vi "FGGA Serial Data Server & Recordingv3.1(serial_sim).vi"() -> ()   [LabVIEW 2014]
uses:
  <vilib>/Platform/TimedLoop/XDataNode/timing_clust.ctl
  <vilib>/Platform/TimedLoop/XDataNode/nitl_modes.ctl
  <vilib>/Platform/TimedLoop/XDataNode/wakeup.ctl
  C:/Program Files (x86)/National Instruments/LabVIEW 2014/examples/Data Communication/Network Streams/Simple Network Streams/support/Network Stream Command.ctl
  <vilib>/Utility/error.llb/whitespace.ctl
  <vilib>/Utility/tcp.llb/UDP Multicast Write-Only Open.vi
  <vilib>/Utility/tcp.llb/UDP Multicast Read-Only Open.vi
  <vilib>/Instr/_visa.llb/VISA Configure Serial Port (Instr).vi
  <vilib>/platform/TimedLoop/XDataNode/XDataNode.xnode
  <vilib>/Platform/TimedLoop/XDataNode/XDNodeRunTimeDep.lvlib
  <vilib>/Instr/_visa.llb/VISA Set IO Buffer Mask.ctl
  <vilib>/Instr/_visa.llb/VISA Flush IO Buffer Mask.ctl
panel:
  out "MFC":dbl[](array[numeric])
  out "FGGA restart":bool
  out "V4":bool
  out "V3":bool
  out "V2":bool
  out "V1":bool
  out "error out 2":errorcluster
  out "error out":errorcluster
  in  "MFC_1 SLPM set value":dbl
  out "Value Read":string
  out "status":bool
  in  "VISA resource name":refnum<visa-resource-name>="ASRL3::INSTR"
  in  "timeout (10sec) 2":u32=3000
  out "Labview_Viewer_UDP_Error_Out":errorcluster
  in  "Clear Display\nErrors":bool
  out "Data Processing":bool
  out "TCP Binary Packet":string
  in  "Time Stamp\nOffset":u32=1
  out "Data String":string
  out "UDP_ACSII_Out":string
  out "Serial error out":errorcluster
  out "SEPTIC TCP Error Out":errorcluster
  out "TCP packet\nSend To SEPTIC":bool
  out "FISH TCP Error Out":errorcluster
  out "TCP packet\nSend To FISH":bool
  out "UDP_Pack_num":u32
  out "UDP_Out Status":bool
  out "UDP_Out_Error Out":errorcluster
  out "UDP_In":string
  out "UDP_In_Error":errorcluster
  in  "Flight Number":string
  out "Data Array":string[](array[string])
  out "RAW DATA":string
  in  "stop":bool
  in  "timeout (10sec)":u32=1500
  in  "VISA resource name":refnum<visa-resource-name>="ASRL7::INSTR"
  out "Number of times \nRead time out":u32
  out "Loop count":i32
  # "Date"
  # "Time"
  # "CH4"
  # "CO2"
  # "H2O"
  # "Cell Pressure"
  # "Cell Temperature"
  # "Spectral Flag"
  # "Ring Down Time (Laser A)"
  # "Ring Down Time (Laser B)"
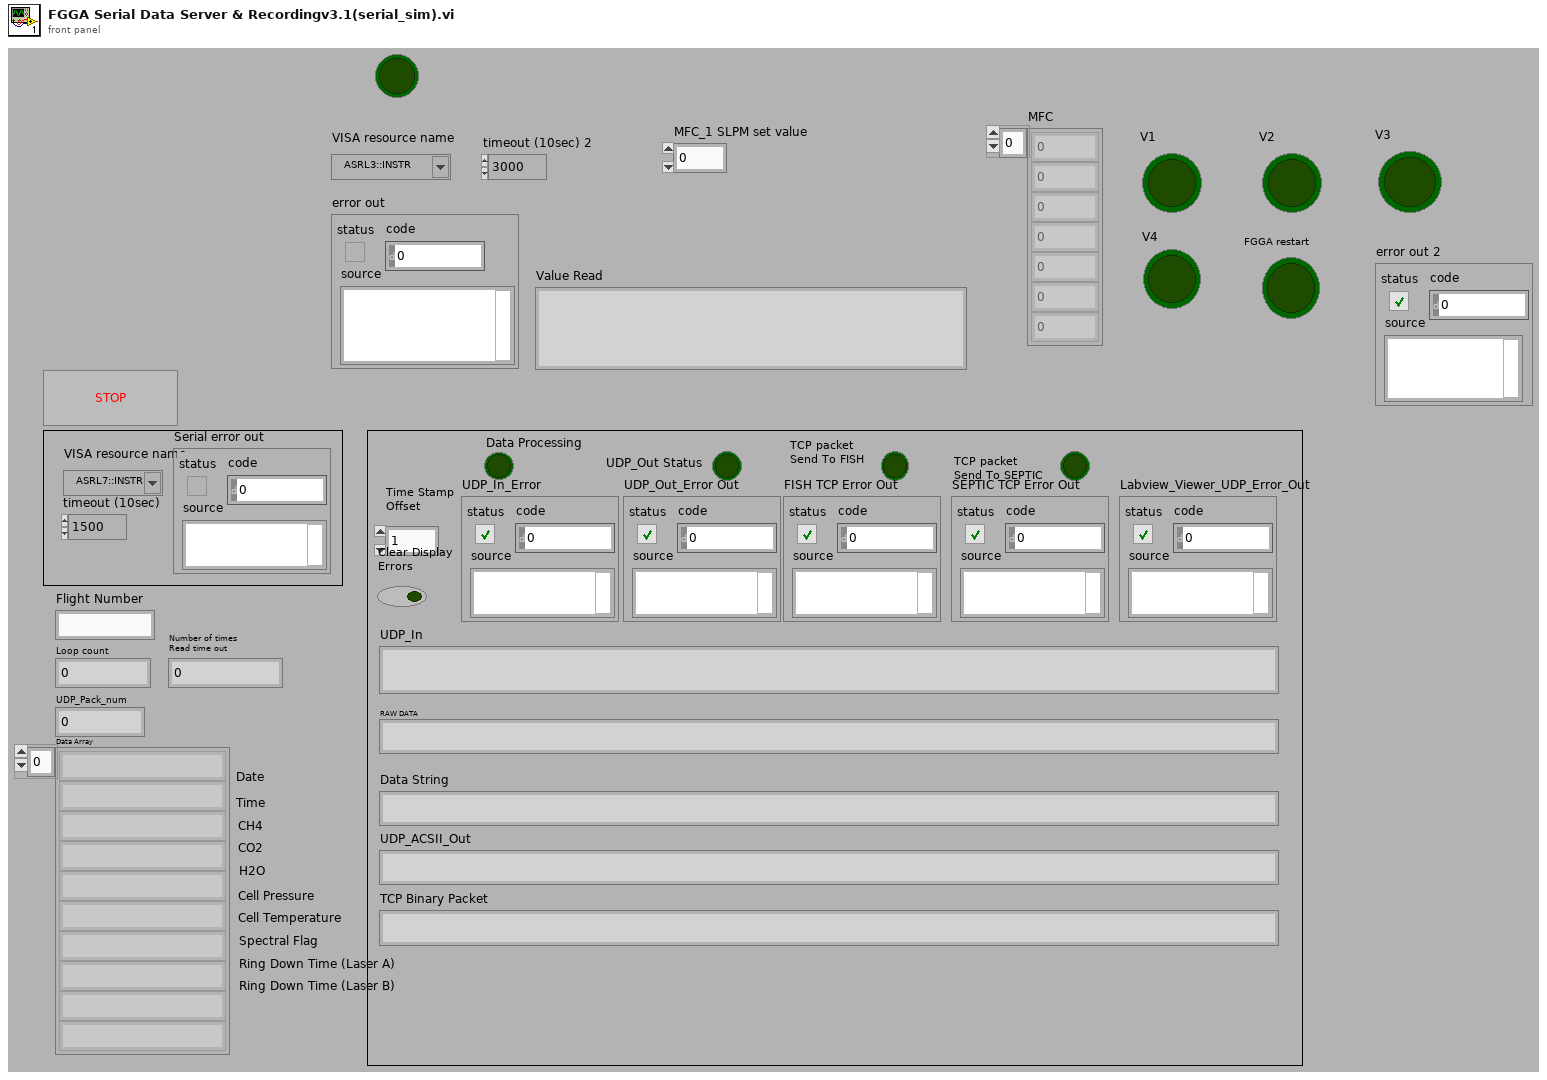
[diagram p1: front panel]
types:
  T1 = typedef "VISA Flush IO Buffer Mask.ctl" = u16
  T2 = typedef "VISA Set IO Buffer Mask.ctl" = u16
  T3 = typedef "Network Stream Command.ctl" = cluster{"Message":string, "Message Data":variant}
  T4 = typedef "XDNodeRunTimeDep.lvlib/timing_clust.ctl" = cluster{"Expected End [f-1]":u64, "Actual End [f-1]":u64, "Finished Late? [f-1]":bool, "Expected End [i-1]":u64, "Actual End [i-1]":u64, "Finished Late? [i-1]":bool, "Expected Start [i]":u64, "Actual Start [i]":u64, "Expected Start [f]":u64, "Actual Start [f]":u64, "Source Name":string, "Structure Name":string, "Period":i64, "Deadline":i64, "Offset":i64, "Start":i64, "Priority":i32, "Timeout":i32, "Mode":T5, "Wakeup Reason":T6, "Error":errorcluster, "Source Type":string, "Secondary Source Type":string, "Global End Time":u64, "Global Start Time":u64, "Frame Duration":u64, "Iteration Duration":u64, "Assigned CPU":i32, "I/O Scan Engine Mode":u32}
  T5 = typedef "XDNodeRunTimeDep.lvlib/nitl_modes.ctl" = enum32{"No Change", "Process missed periods, maintain original phase", "Discard missed periods, maintain original phase", "Process missed periods, ignore original phase", "Discard missed periods, ignore original phase"}
  T6 = typedef "XDNodeRunTimeDep.lvlib/wakeup.ctl" = enum32{"Normal", "Aborted", "Asynchronous wakeup", "Timing source error", "Timed loop error", "Timeout"}
  T7 = typedef "whitespace.ctl" = u16
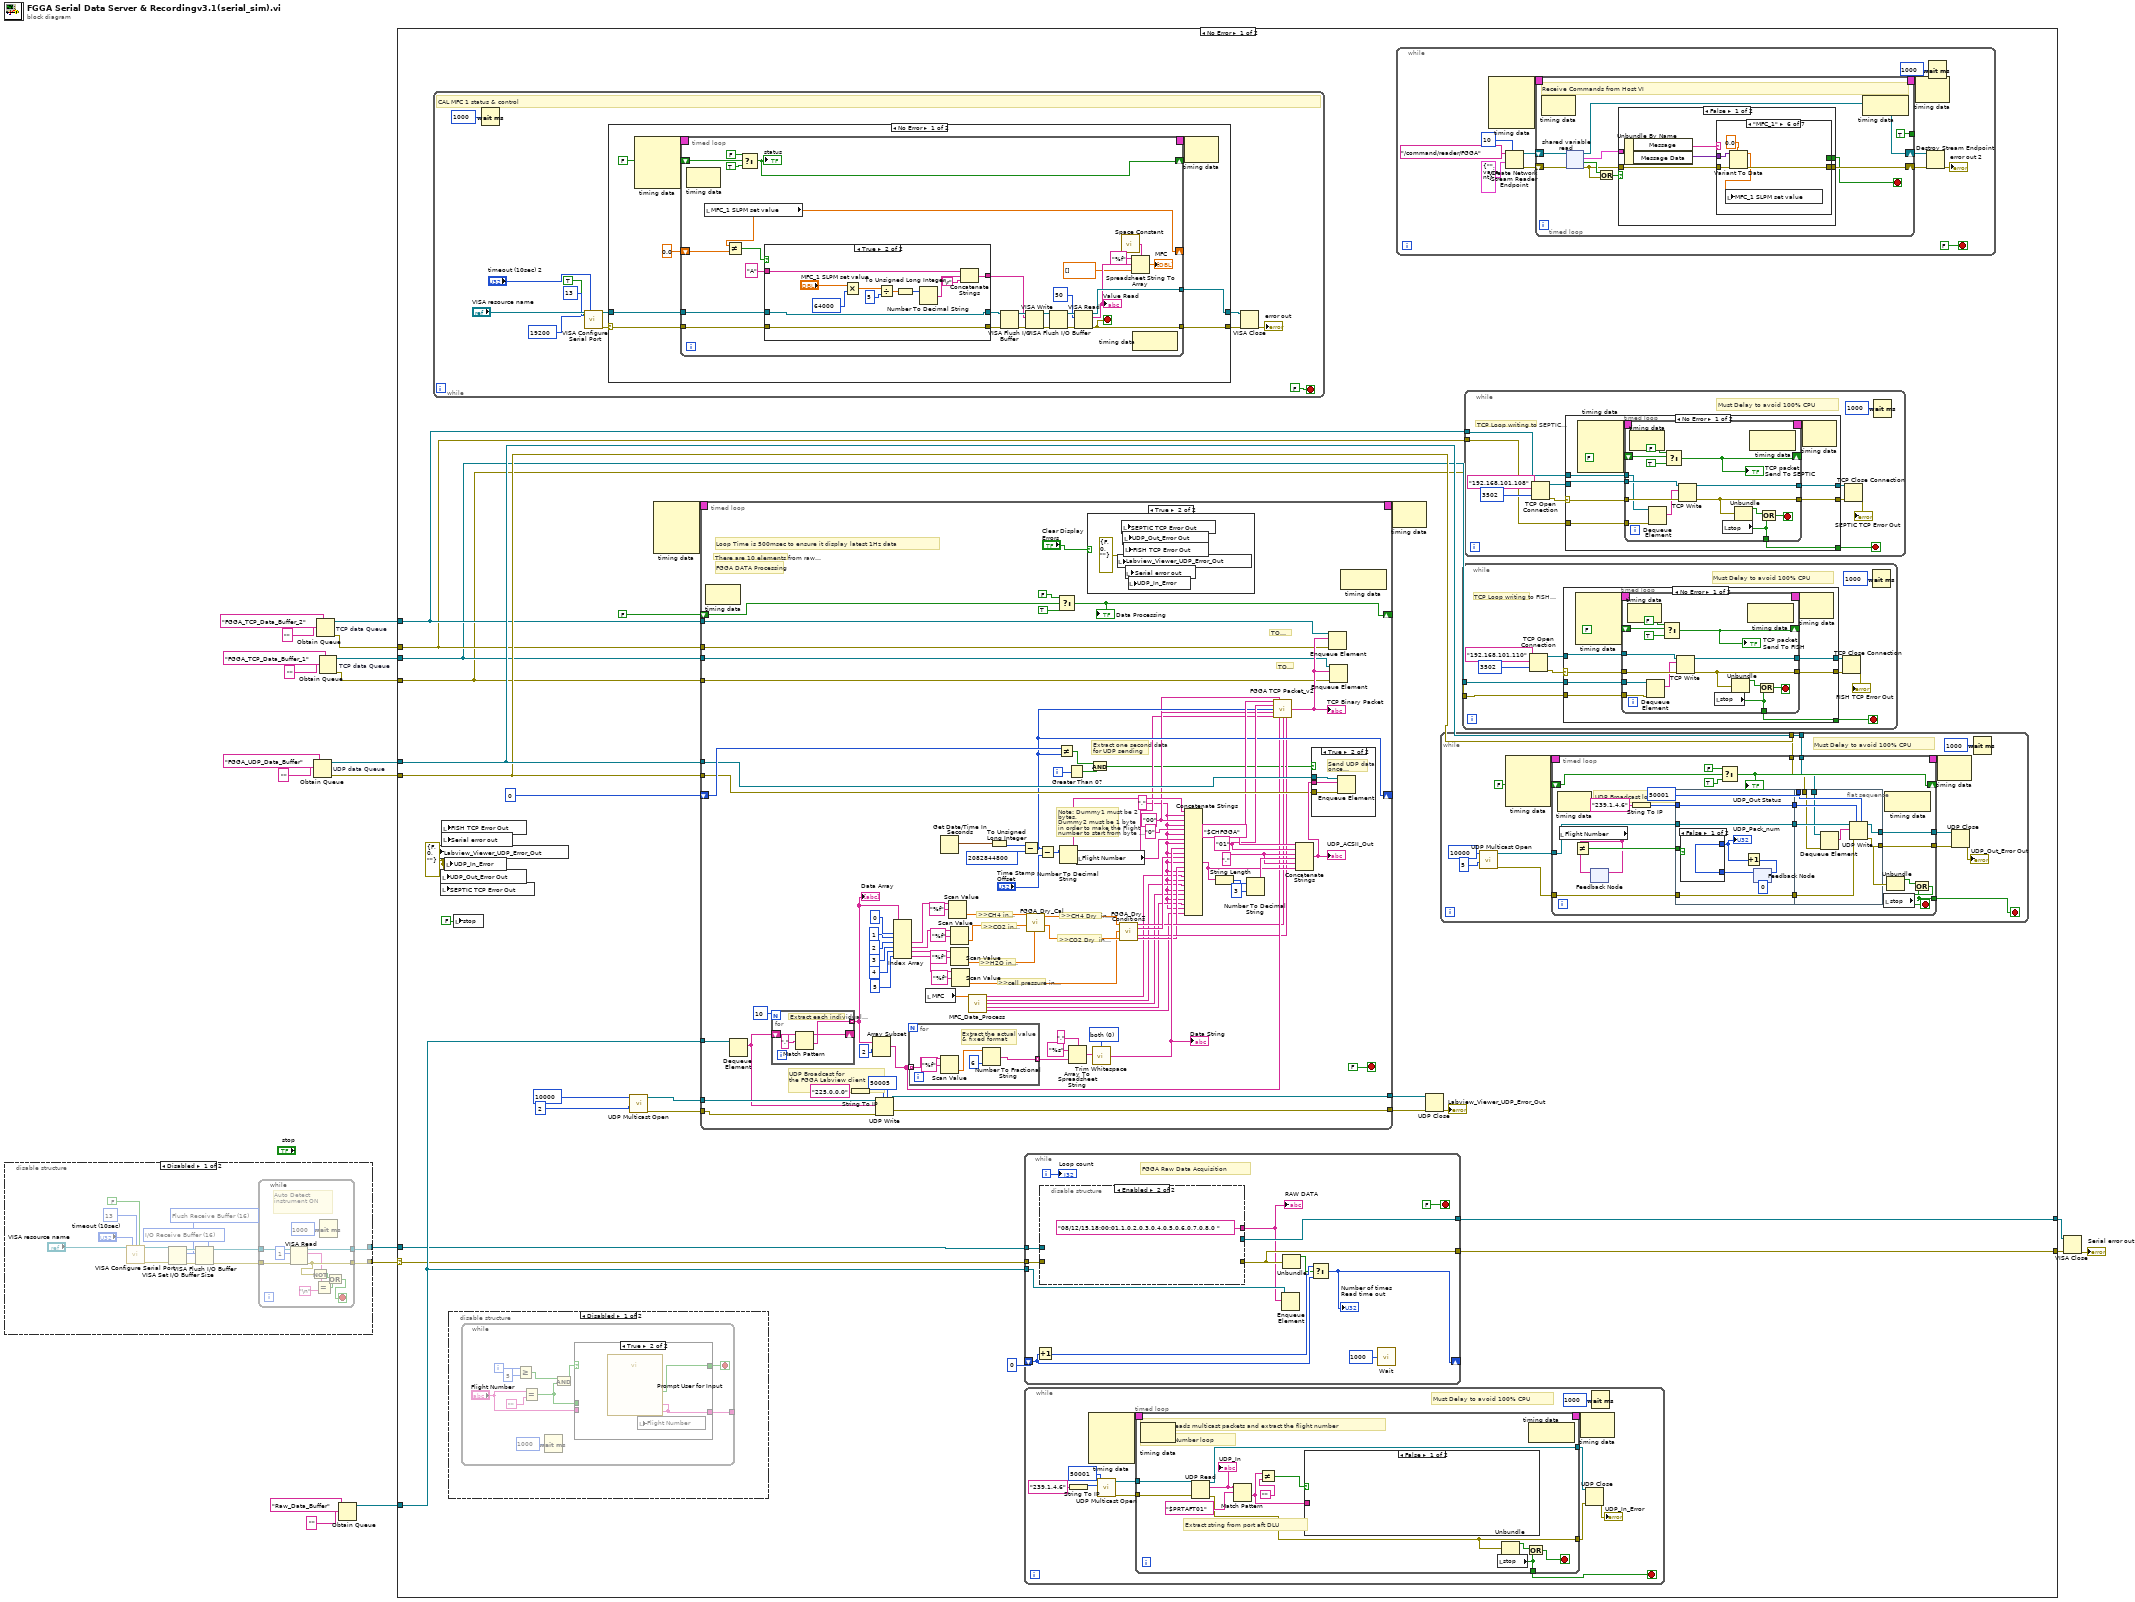
[diagram p0: block diagram]
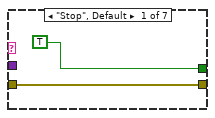
[diagram p3: hidden frame]
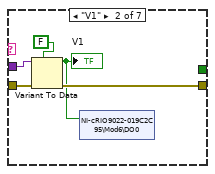
[diagram p4: hidden frame]
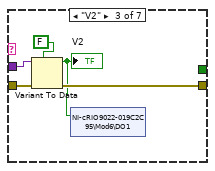
[diagram p5: hidden frame]
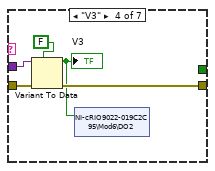
[diagram p6: hidden frame]
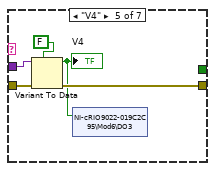
[diagram p7: hidden frame]
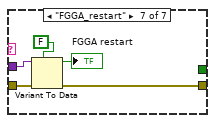
[diagram p8: hidden frame]
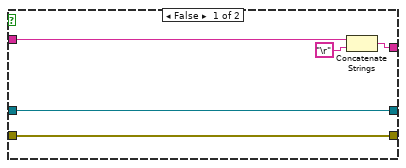
[diagram p10: hidden frame]
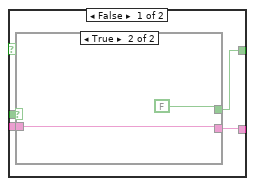
[diagram p12: hidden frame]
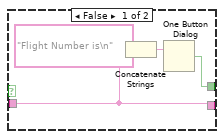
[diagram p13: hidden frame]
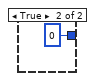
[diagram p15: hidden frame]
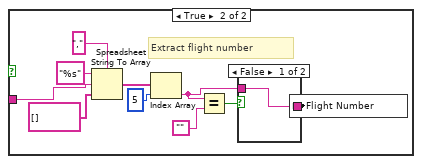
[diagram p16: hidden frame]
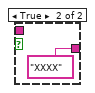
[diagram p17: hidden frame]
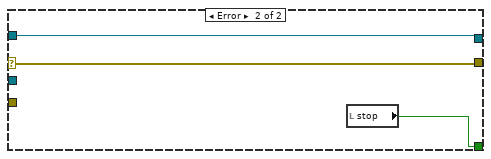
[diagram p18: hidden frame]
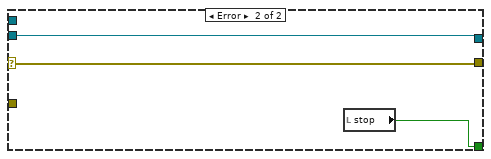
[diagram p19: hidden frame]
diagram:
  n1 = disable-structure shown="Disabled" {
    disable-tunnel: [w22 _] -> w2
    disable-tunnel: [w21 _] -> w1
    frame Disabled {
      w27 = T1 16 items=["Flush Receive Buffer"=16, "Write Transmit Buffer to Device"=32, "Flush Receive Buffer (No I/O)"=64, "Flush Transmit Buffer"=128] ("Mask")
      w28 = T2 16 items=["I/O Receive Buffer"=16, "I/O Transmit Buffer"=32, "I/O Receive and Transmit Buffer"=48] ("Mask")
      n2 = call-poly "VISA Configure Serial Port"("VISA resource name"="VISA resource name", "timeout (10sec)"="timeout (10sec)", "termination char\n(0xA = '\\n' = LF)"=u8 13 ("termination char\n(0xA = '\\n' = LF)"), "Enable Termination\nChar (T)"=FALSE ("Enable Termination\nChar (T)")) -> ("VISA resource name out"=w26:refnum<visa-resource-name>, "error out"=w25:errorcluster)  [unwired: 10 in]
      n3 = VISA Set I/O Buffer Size(VISA resource name=w26, mask (16)=w28, error in (no error)=w25) -> (VISA resource name out=w29:refnum<visa-resource-name>, error out=w30:errorcluster)  [unwired: 1 in]
      n4 = VISA Flush I/O Buffer(VISA resource name=w29, mask (16)=w27, error in (no error)=w30) -> (VISA resource name out=w24:refnum<visa-resource-name>, error out=w23:errorcluster)
      n5 = while {
        tunnel: w24 -> [w45]
        tunnel: w23 -> [w44]
        tunnel: [w42] -> w22
        tunnel: [w41] -> w21
        stop <- w36 stop-if-true
        # "Auto Detect\ninstrument ON"
        n6 = VISA Read(VISA resource name=w45, byte count=u32 1, error in (no error)=w44) -> (VISA resource name out=w41:refnum<visa-resource-name>, read buffer=w39:string, error out=w42:errorcluster)  [unwired: 1 out]
        n7 = Not(x=w42) -> (.not. x?=w38:bool)
        n8 = Equal?(x=w39, y="\n") -> (x = y?=w37:bool)
        n9 = Wait (ms)(milliseconds to wait=u32 1000) -> ()  [unwired: 1 out]
        n10 = Or(x=w38, y=w37) -> (x .or. y?=w36:bool)
      }
    }
    frame Enabled {
    }
  }
  n11 = Obtain Queue "UDP data Queue"(name (unnamed)="FGGA_UDP_Data_Buffer", element data type="") -> (queue out=w12:refnum<queue>, error out=w11:errorcluster)  [unwired: 3 in, 1 out]
  n12 = Obtain Queue "TCP data Queue"(name (unnamed)="FGGA_TCP_Data_Buffer_2", element data type="") -> (queue out=w6:refnum<queue>, error out=w5:errorcluster)  [unwired: 3 in, 1 out]
  n13 = Obtain Queue "TCP data Queue"(name (unnamed)="FGGA_TCP_Data_Buffer_1", element data type="") -> (queue out=w4:refnum<queue>, error out=w3:errorcluster)  [unwired: 3 in, 1 out]
  n14 = Obtain Queue(name (unnamed)="Raw_Data_Buffer", element data type="") -> (queue out=w18:refnum<queue>)  [unwired: 3 in, 2 out]
  n15 = case shown="No Error" w2 {
    selector: w2 -> [w46 w545]
    tunnel: w1 -> [w47 w546]
    tunnel: [w69 w546] -> w15
    tunnel: [w70 w545] -> w16
    tunnel: w18 -> [w65 _]
    tunnel: w12 -> [w63 _]
    tunnel: w11 -> [w62 _]
    tunnel: w6 -> [w61 _]
    tunnel: w5 -> [w60 _]
    tunnel: w4 -> [w59 _]
    tunnel: w3 -> [w58 _]
    frame No Error {
      w49 = errorcluster {"status"=FALSE, "code"=0, "source"=""} ("UDP Error Out")
      n16 = while {
        stop <- FALSE stop-if-true
        # "CAL MFC 1 status & control"
        n17 = Wait (ms)(milliseconds to wait=u32 1000) -> ()  [unwired: 1 out]
        n18 = call-poly "VISA Configure Serial Port"("VISA resource name"="VISA resource name", "timeout (10sec)"="timeout (10sec) 2", "termination char\n(0xA = '\\n' = LF)"=u8 13 ("termination char\n(0xA = '\\n' = LF)"), "Enable Termination\nChar (T)"=TRUE ("Enable Termination\nChar (T)"), "baud rate (9600)"=u32 19200) -> ("VISA resource name out"=w148:refnum<visa-resource-name>, "error out"=w144:errorcluster)  [unwired: 9 in]
        n19 = case shown="No Error" w144 {
          selector: w144 -> [w155 w205]
          tunnel: w148 -> [w156 w206]
          tunnel: [w154 w206] -> w147
          tunnel: [w153 w205] -> w146
          frame No Error {
            n20 = node-c288() -> (w151:T4)  [unwired: 4 in]
            n21 = timed-loop {
              tunnel: w156 -> [w179]
              tunnel: w155 -> [w177]
              tunnel: [w170] -> w154
              tunnel: [w165] -> w153
              shift-right: [w166] -> _
              shift-left: FALSE -> [w169]
              timing: w151 -> [_]
              timing-out: [_] -> w150
              shift-right: [w157] -> _
              shift-left: 0.0 -> [w159]
              stop <- w165 stop-if-true
              n22 = node-c288() -> ()  [unwired: 1 in, 1 out]
              n23 = local read "MFC_1 SLPM set value"() -> (w157:dbl)
              n24 = Not Equal?(x=w157, y=w159) -> (x != y?=w158:bool)
              n25 = Select(t=FALSE, s=w169, f=TRUE) -> (s? t:f=w166:bool)
              "status" <- w166
              n26 = case shown="True" w158 {
                tunnel: w179 -> [w187 w202]
                tunnel: [w187 w202] -> w178
                tunnel: w177 -> [w186 w201]
                tunnel: [w186 w201] -> w176
                tunnel: "A" -> [w190 w194]
                tunnel: [w188 w191] -> w174
                frame False {
                  n27 = Concatenate Strings(w190, "\r") -> (w188:string)
                }
                frame True {
                  n28 = Multiply(x="MFC_1 SLPM set value", y=u32 64000) -> (x*y=w198:dbl)
                  n29 = Divide(x=w198, y=u32 5) -> (x/y=w196:dbl)
                  n30 = To Unsigned Long Integer(number=w196) -> (unsigned 32bit integer=w195:u32)
                  n31 = Number To Decimal String(number=w195) -> (decimal integer string=w193:string)  [unwired: 1 in]
                  n32 = Concatenate Strings(w194, w193, "\r") -> (w191:string)
                }
              }
              n33 = VISA Flush I/O Buffer(VISA resource name=w178, error in (no error)=w176) -> (VISA resource name out=w181:refnum<visa-resource-name>, error out=w180:errorcluster)  [unwired: 1 in]
              n34 = VISA Write(VISA resource name=w181, write buffer=w174, error in (no error)=w180) -> (VISA resource name out=w173:refnum<visa-resource-name>, error out=w172:errorcluster)  [unwired: 1 out]
              n35 = VISA Flush I/O Buffer(VISA resource name=w173, error in (no error)=w172) -> (VISA resource name out=w183:refnum<visa-resource-name>, error out=w182:errorcluster)  [unwired: 1 in]
              n36 = VISA Read(VISA resource name=w183, byte count=u32 50, error in (no error)=w182) -> (VISA resource name out=w170:refnum<visa-resource-name>, read buffer=w164:string, error out=w165:errorcluster)  [unwired: 1 out]
              "Value Read" <- w164
              n37 = call <vilib>:"Space Constant.vi"() -> ("String"=w163:string)
              n38 = Spreadsheet String To Array(delimiter (Tab)=w163, format string="%f", spreadsheet string=w164, array type (2D Dbl)=dbl[] []) -> (array=→"MFC":dbl[])
              n39 = node-c288() -> ()  [unwired: 1 in, 1 out]
            }
            n40 = node-c288(w150) -> ()  [unwired: 1 out]
          }
          frame Error {
          }
        }
        n41 = VISA Close(VISA resource name=w147, error in (no error)=w146) -> (error out=→"error out":errorcluster)
      }
      n42 = local write "Labview_Viewer_UDP_Error_Out"(w49) -> ()
      n43 = local write "UDP_Out_Error Out"(w49) -> ()
      n44 = local write "SEPTIC TCP Error Out"(w49) -> ()
      n45 = local write "FISH TCP Error Out"(w49) -> ()
      n46 = local write "Serial error out"(w49) -> ()
      n47 = local write "UDP_In_Error"(w49) -> ()
      n48 = disable-structure shown="Disabled" {
        frame Disabled {
          n49 = while {
            tunnel: [w213] -> _
            i -> [w212]
            stop <- w215 stop-if-true
            n50 = Greater Or Equal?(x=w212, y=5) -> (x >= y?=w210:bool)
            n51 = Equal?(x="Flight Number", y="") -> (x = y?=w208:bool)
            n52 = Wait (ms)(milliseconds to wait=u32 1000) -> ()  [unwired: 1 out]
            n53 = And(x=w210, y=w208) -> (x .and. y?=w209:bool)
            n54 = case shown="True" w209 {
              tunnel: [w217 w228] -> w215
              tunnel: [w218 w227] -> w213
              tunnel: w208 -> [w220 _]
              tunnel: "Flight Number" -> [w219 _]
              frame False {
                n55 = case shown="True" w220 {
                  tunnel: [w222 w226] -> w218
                  tunnel: w219 -> [w222 w226]
                  tunnel: [w224 FALSE] -> w217
                  frame False {
                    n56 = Concatenate Strings("Flight Number is\n" ("string"), w222) -> (w221:string)
                    n57 = One Button Dialog(message=w221) -> (true=w224:bool)  [unwired: 1 in]
                  }
                  frame True {
                  }
                }
              }
              frame True {
                n58 = call "Prompt User for Input"() -> ("Flight Number BXXX"=w227:string, "OK"=w228:bool)  [unwired: 17 in, 1 out]
                n59 = local write "Flight Number"(w227) -> ()
              }
            }
          }
        }
        frame Enabled {
        }
      }
      n60 = local write "stop"(FALSE ("stop")) -> ()
      n61 = call-poly <vilib>:"UDP Multicast Open.vi"("time-to-live (1)"=u16 2, "port"=u16 10000) -> ("error out"=w53:errorcluster, "connection ID"=w54:refnum<k16>)  [unwired: 8 in]
      n62 = node-c288() -> (w67:T4)  [unwired: 4 in]
      n63 = timed-loop {
        timing: w67 -> [_]
        timing-out: [_] -> w66
        tunnel: w65 -> [w497]
        tunnel: w63 -> [w458]
        tunnel: w62 -> [w457]
        shift-right: [w454] -> _
        shift-left: u32 0 -> [w461]
        tunnel: w61 -> [w449]
        tunnel: w60 -> [w448]
        tunnel: w59 -> [w447]
        tunnel: w58 -> [w446]
        shift-right: [w442] -> _
        shift-left: FALSE -> [w445]
        tunnel: w54 -> [w438]
        tunnel: w53 -> [w437]
        tunnel: [w436] -> w52
        tunnel: [w435] -> w51
        i -> [w460]
        stop <- FALSE stop-if-true
        w453 = "00"
        w415 = ","
        w483 = T7 0 items=["both", "start of string", "end of string"] ("location (both)")
        w491 = ","
        w455 = "01"
        w456 = "$CHFGGA"
        # "Note: Dummy1 must be 2 bytes, \nDummy2 must be 1 byte\nin order to make the Flight \nnumber to start from byte 20\n(this only applies to TCP packet)"
        # ">>cell pressure in torr>>"
        # "UDP Broadcast for\nthe FGGA Labview client"
        # "There are 10 elements from raw packet"
        # "TO SEPTIC"
        # "TO FISH"
        # "Extract one second data\nfor UDP sending"
        # ">>CO2 Dry  in ppm>>"
        # ">>CH4 Dry  in ppb>>"
        # ">>H2O in ppm>>"
        # ">>CO2 in ppm>>"
        # ">>CH4 in ppm>>"
        # "Loop Time is 500msec to ensure it display latest 1Hz data"
        # "FGGA DATA Processing"
        n64 = node-c288() -> ()  [unwired: 1 in, 1 out]
        n65 = Dequeue Element(queue=w497) -> (element=w434:string)  [unwired: 2 in, 3 out]
        n66 = for {
          N: 10 -> [_]
          shift-right: [w509] -> _
          shift-left: w434 -> [w507]
          tunnel: [w508] -> w488 mode=indexing
          # "Extract each individual param"
          n67 = Match Pattern(string=w507, regular expression=",") -> (before substring=w508:string, after substring=w509:string)  [unwired: 1 in, 2 out]
        }
        "Data Array" <- w488
        n68 = String To IP(1:"225.0.0.0" ("name")) -> (0:w439:u32)
        n69 = Array Subset(array=w488, index=2) -> (w451:string[])  [unwired: 1 in]
        n70 = UDP Write(address=w439, port or service name=u16 50005, connection ID=w438, data in=w434, 8:w437) -> (error out=w435:errorcluster, 3:w436:refnum<k16>)  [unwired: 1 in]
        n71 = Index Array(array=w488, index #1=0 ("index"), index #2=1 ("index"), index #3=2 ("index"), index #4=3 ("index"), index #5=4 ("index"), index #6=5 ("index")) -> (element #3=w471:string, element #4=w470:string, element #5=w469:string, element #6=w425:string)  [unwired: 2 out]
        n72 = for {
          tunnel: w451 -> [w505] mode=indexing
          tunnel: [w502] -> w481 mode=indexing
          # "Extract the actual value\n& fixed format"
          n73 = Scan Value(string=w505, format string="%f") -> (value=w503:dbl)  [unwired: 1 in, 1 out]
          n74 = Number To Fractional String(number=w503, precision (6)=i16 6) -> (F-format string=w502:string)  [unwired: 2 in]
        }
        n75 = local read "MFC"() -> (w420:dbl[])
        n76 = Get Date/Time In Seconds() -> (seconds since 1Jan1904=w412:timestamp)
        n77 = Scan Value(string=w471, format string="%f") -> (value=w473:dbl)  [unwired: 1 in, 1 out]
        n78 = Scan Value(string=w470, format string="%f") -> (value=w472:dbl)  [unwired: 1 in, 1 out]
        n79 = Scan Value(string=w469, format string="%f") -> (value=w422:dbl)  [unwired: 1 in, 1 out]
        n80 = Scan Value(string=w425, format string="%f") -> (value=w423:dbl)  [unwired: 1 in, 1 out]
        n81 = call "MFC_Data_Process.vi"("MFC"=w420) -> ("MFC Absolute Pressure"=w419:string, "MFC Temperature"=w418:string, "MFC Volumetric Flow"=w417:string, "MFC Mass Flow"=w416:string, "MFC Set Point"=w414:string)  [unwired: 10 in]
        n82 = To Unsigned Long Integer(number=w412) -> (unsigned 32bit integer=w467:u32)
        n83 = Subtract(x=w467, y=u32 2082844800) -> (x-y=w454:u32)
        n84 = call "FGGA_Dry_Cal.vi"("H2O"=w422, "CO2_Wet"=w472, "CH4_Wet"=w473) -> ("CO2_Dry"=w427:dbl, "CH4_Dry"=w429:dbl)  [unwired: 7 in]
        n85 = Subtract(x=w454, y="Time Stamp\nOffset") -> (x-y=w464:u32)
        n86 = Select(t=FALSE, s=w445, f=TRUE) -> (s? t:f=w442:bool)
        "Data Processing" <- w442
        n87 = Not Equal?(x=w461, y=w454) -> (x != y?=w462:bool)
        n88 = Number To Decimal String(number=w464) -> (decimal integer string=w466:string)  [unwired: 1 in]
        n89 = Greater Than 0?(x=w460) -> (x > 0?=w463:bool)
        n90 = Array To Spreadsheet String(delimiter (Tab)=",", array=w481, 3:"%s" ("format string")) -> (spreadsheet string=w482:string)
        n91 = local read "Flight Number"() -> (w452:string)
        n92 = case shown="True" "Clear Display\nErrors" {
          frame False {
          }
          frame True {
            w498 = errorcluster {"status"=FALSE, "code"=0, "source"=""} ("UDP Error Out")
            n93 = local write "Labview_Viewer_UDP_Error_Out"(w498) -> ()
            n94 = local write "SEPTIC TCP Error Out"(w498) -> ()
            n95 = local write "UDP_Out_Error Out"(w498) -> ()
            n96 = local write "FISH TCP Error Out"(w498) -> ()
            n97 = local write "Serial error out"(w498) -> ()
            n98 = local write "UDP_In_Error"(w498) -> ()
          }
        }
        n99 = call <vilib>:"Trim Whitespace.vi"("string"=w482, "location (both)"=w483) -> ("trimmed string"=w480:string)
        "Data String" <- w480
        n100 = Compound Arithmetic op=AND(w462, w463) -> (w413:bool)
        n101 = call "FGGA_Dry_Conditions.vi"("CH4_Dry"=w429, "Pressure"=w423, "CO2_Dry"=w427) -> ("CH4_Dry_TCP"=w432:string, "CH4_Dry_UDP"=w433:string, "CO2_Dry_TCP"=w431:string, "CO2_Dry_UDP"=w430:string)  [unwired: 9 in]
        n102 = Concatenate Strings(w466, w415, w453, w415, "0" ("string"), w415, w452, w415, w480, w415, w433, w415, w430, w415, w419, w415, w418, w415, w417, w415, w416, w415, w414) -> (w490:string)
        n103 = String Length(string=w490) -> (length=w494:i32)
        n104 = Number To Decimal String(number=w494, width (-)=i16 3) -> (decimal integer string=w492:string)
        n105 = call "FGGA TCP Packet_v2.vi"("ID"=w456, "dummy2"=w453, "Version"=w455, "utc_time"=w454, "dummy1"=w453, "Flight Number"=w452, "Data Array"=w451, "ch4_dry"=w432, "co2_dry"=w431) -> ("TCP Binary Packet"=w450:string)  [unwired: 6 in]
        "TCP Binary Packet" <- w450
        n106 = Concatenate Strings(w456, w455, w491, w492, w491, w490) -> (w459:string)
        "UDP_ACSII_Out" <- w459
        n107 = case shown="True" w413 {
          tunnel: w459 -> [_ w501]
          tunnel: w458 -> [_ w500]
          tunnel: w457 -> [_ w499]
          frame False {
          }
          frame True {
            # "Send UDP data once\na second"
            n108 = Enqueue Element(queue=w500, element=w501, error in (no error)=w499) -> ()  [unwired: 1 in, 3 out]
          }
        }
        n109 = Enqueue Element(queue=w449, element=w450, error in (no error)=w448) -> ()  [unwired: 1 in, 3 out]
        n110 = Enqueue Element(queue=w447, element=w450, error in (no error)=w446) -> ()  [unwired: 1 in, 3 out]
        n111 = node-c288() -> ()  [unwired: 1 in, 1 out]
      }
      n112 = while {
        tunnel: w47 -> [w527]
        tunnel: w46 -> [w526]
        tunnel: [w525] -> w70
        shift-right: [w521] -> _
        shift-left: u32 0 -> [w522]
        tunnel: [w524] -> w69
        tunnel: w65 -> [w519]
        i -> [w523]
        stop <- FALSE stop-if-true
        # "FGGA Raw Data Acquisition"
        n113 = Increment(x=w522) -> (x+1=w520:u32)
        n114 = disable-structure shown="Enabled" {
          disable-tunnel: w527 -> [w533 _]
          disable-tunnel: w526 -> [w532 _]
          disable-tunnel: [w531 _] -> w525
          disable-tunnel: [w530 _] -> w524
          disable-tunnel: [w528 "08/12/15,18:00:01,1.0,2.0,3.0,4.0,5.0,6.0,7.0,8.0 " ("RAW DATA")] -> w518
          frame Disabled {
            n115 = while {
              tunnel: [w543] -> w530
              tunnel: [w542] -> w531
              tunnel: w533 -> [w541]
              tunnel: w532 -> [w540]
              shift-right: [w538] -> w528
              shift-left: "" -> [w539]
              stop <- w535 stop-if-true
              # "Read 1 byte at a time \nuntil line feed is reached"
              n116 = VISA Read(VISA resource name=w541, byte count=u32 1, error in (no error)=w540) -> (VISA resource name out=w543:refnum<visa-resource-name>, read buffer=w537:string, error out=w542:errorcluster)  [unwired: 1 out]
              n117 = Concatenate Strings(w539, w537) -> (w538:string)
              n118 = Equal?(x=w537, y="\n") -> (x = y?=w535:bool)
            }
          }
          frame Enabled {
          }
        }
        "RAW DATA" <- w518
        n119 = Enqueue Element(queue=w519, element=w518) -> ()  [unwired: 2 in, 3 out]
        n120 = Unbundle(w525) -> ("status"=w517:bool)  [unwired: 2 out]
        n121 = Select(t=w520, s=w517, f=w522) -> (s? t:f=w521:u32)
        "Number of times \nRead time out" <- w521
        n122 = call "Wait"("Count(mSec)"=u32 1000) -> ()  [unwired: 1 out]
        "Loop count" <- w523
      }
      n123 = while {
        stop <- w289 stop-if-true
        # "Must Delay to avoid 100% CPU"
        n124 = String To IP(1:"239.1.4.6" ("name")) -> (0:w297:u32)
        n125 = node-c288() -> (w299:T4)  [unwired: 4 in]
        n126 = call-poly <vilib>:"UDP Multicast Open.vi"("multicast addr"=w297, "port"=u16 50001) -> ("error out"=w293:errorcluster, "connection ID"=w294:refnum<k16>)  [unwired: 7 in, 1 out]
        n127 = timed-loop {
          tunnel: w294 -> [w311]
          tunnel: w293 -> [w310]
          timing: w299 -> [_]
          timing-out: [_] -> w298
          tunnel: [w304] -> w291
          tunnel: [w302] -> w290
          tunnel: [w300] -> w289
          stop <- w301 stop-if-true
          # "Extract string from port aft DLU"
          # "Get Flight Number loop"
          # "This loop reads multicast packets and extract the flight number"
          n128 = node-c288() -> ()  [unwired: 1 in, 1 out]
          n129 = UDP Read(connection ID=w311, 8:w310) -> (data out=w309:string, error out=w302:errorcluster, 3:w304:refnum<k16>)  [unwired: 2 in, 2 out]
          "UDP_In" <- w309
          n130 = Match Pattern(string=w309, regular expression="$PRTAFT01") -> (after substring=w305:string)  [unwired: 1 in, 3 out]
          n131 = Not Equal?(x=w305, y="") -> (x != y?=w306:bool)
          n132 = case shown="False" w306 {
            tunnel: w305 -> [_ w318]
            frame False {
            }
            frame True {
              # "Extract flight number"
              n133 = Spreadsheet String To Array(delimiter (Tab)=",", format string="%s", spreadsheet string=w318, array type (2D Dbl)=string[] []) -> (array=w320:string[])
              n134 = Index Array(array=w320, index=5) -> (element=w314:string)
              n135 = Equal?(x=w314, y="") -> (x = y?=w317:bool)
              n136 = case shown="False" w317 {
                tunnel: [w324 "XXXX"] -> w315
                tunnel: w314 -> [w324 _]
                frame False {
                }
                frame True {
                }
              }
              n137 = local write "Flight Number"(w315) -> ()
            }
          }
          n138 = local read "stop"() -> (w300:bool)
          n139 = Unbundle(w302) -> ("status"=w303:bool)  [unwired: 2 out]
          n140 = node-c288() -> ()  [unwired: 1 in, 1 out]
          n141 = Compound Arithmetic op=OR(w303, w300) -> (w301:bool)
        }
        n142 = node-c288(w298) -> ()  [unwired: 1 out]
        n143 = UDP Close(connection ID=w291, 8:w290) -> (error out=→"UDP_In_Error":errorcluster)  [unwired: 1 out]
        n144 = Wait (ms)(milliseconds to wait=u32 1000) -> ()  [unwired: 1 out]
      }
      n145 = node-c288(w66) -> ()  [unwired: 1 out]
      n146 = while {
        stop <- FALSE stop-if-true
        n147 = node-c288() -> (w72:T4)  [unwired: 4 in]
        n148 = Create Network Stream Reader Endpoint(7:10 ("reader buffer size"), 9:T3 {"Message"="", "Message Data"=variant} ("Message Cluster"), 11:"/command/reader/FGGA" ("reader url")) -> (0:w78:errorcluster, 3:w79:refnum<k21>)  [unwired: 4 in]
        n149 = timed-loop "Host->Target Command Reader" {
          shift-right: [w89] -> w76
          shift-left: w78 -> [w92]
          shift-right: [w90] -> w75
          shift-left: w79 -> [w91]
          tunnel: [TRUE] -> _
          timing: w72 -> [_]
          timing-out: [_] -> w71
          stop <- w83 stop-if-true
          # "Receive Commands from Host VI"
          n150 = node-c288() -> ()  [unwired: 1 in, 1 out]
          n151 = shared-variable-read(w91, w92) -> (w90:refnum<k21>, w85:errorcluster, w87:bool, w88:T3)  [unwired: 1 in]
          n152 = Or(x=w87, y=w85) -> (x .or. y?=w86:bool)
          n153 = case shown="False" w86 {
            selector: w86 -> [_ w133]
            tunnel: w85 -> [w100 w134]
            tunnel: [w99 w134] -> w89
            tunnel: w88 -> [w97 _]
            tunnel: [w98 w133] -> w83
            frame False {
              n154 = Unbundle By Name(w97) -> ("Message"=w96:string, "Message Data"=w95:variant)
              n155 = case shown="\"MFC_1\"" w96 {
                tunnel: w100 -> [w102 w107 w112 w117 w122 w127 w132]
                tunnel: [w102 w106 w111 w116 w121 w126 w131] -> w99
                tunnel: w95 -> [_ w105 w110 w115 w120 w125 w130]
                tunnel: [TRUE _ _ _ _ _ _] -> w98
                frame "Stop", Default {
                }
                frame "V1" {
                  n156 = Variant To Data(error in=w107, type=FALSE, Variant=w105) -> (data=w103:bool, error out=w106:errorcluster)
                  "V1" <- w103
                  n157 = shared-variable "NI-cRIO9022-019C2C95\\Mod6\\DO0"(w103) -> ()  [unwired: 1 in, 1 out]
                }
                frame "V2" {
                  n158 = Variant To Data(error in=w112, type=FALSE, Variant=w110) -> (data=w108:bool, error out=w111:errorcluster)
                  "V2" <- w108
                  n159 = shared-variable "NI-cRIO9022-019C2C95\\Mod6\\DO1"(w108) -> ()  [unwired: 1 in, 1 out]
                }
                frame "V3" {
                  n160 = Variant To Data(error in=w117, type=FALSE, Variant=w115) -> (data=w113:bool, error out=w116:errorcluster)
                  "V3" <- w113
                  n161 = shared-variable "NI-cRIO9022-019C2C95\\Mod6\\DO2"(w113) -> ()  [unwired: 1 in, 1 out]
                }
                frame "V4" {
                  n162 = Variant To Data(error in=w122, type=FALSE, Variant=w120) -> (data=w118:bool, error out=w121:errorcluster)
                  "V4" <- w118
                  n163 = shared-variable "NI-cRIO9022-019C2C95\\Mod6\\DO3"(w118) -> ()  [unwired: 1 in, 1 out]
                }
                frame "MFC_1" {
                  n164 = Variant To Data(error in=w127, type=0.0, Variant=w125) -> (data=w123:dbl, error out=w126:errorcluster)
                  n165 = local write "MFC_1 SLPM set value"(w123) -> ()
                }
                frame "FGGA_restart" {
                  n166 = Variant To Data(error in=w132, type=FALSE, Variant=w130) -> (data=→"FGGA restart":bool, error out=w131:errorcluster)
                }
              }
            }
            frame True {
            }
          }
          n167 = node-c288() -> ()  [unwired: 1 in, 1 out]
        }
        n168 = node-c288(w71) -> ()  [unwired: 1 out]
        n169 = Destroy Stream Endpoint(8:w76, 11:w75) -> (0:→"error out 2":errorcluster)
        n170 = Wait (ms)(milliseconds to wait=u32 1000) -> ()  [unwired: 1 out]
      }
      n171 = UDP Close(connection ID=w52, 8:w51) -> (error out=→"Labview_Viewer_UDP_Error_Out":errorcluster)  [unwired: 1 out]
      n172 = while {
        tunnel: w63 -> [w231]
        tunnel: w62 -> [w230]
        stop <- w232 stop-if-true
        # "Must Delay to avoid 100% CPU"
        n173 = call-poly <vilib>:"UDP Multicast Open.vi"("time-to-live (1)"=u16 5, "port"=u16 10000) -> ("error out"=w239:errorcluster, "connection ID"=w240:refnum<k16>)  [unwired: 8 in]
        n174 = node-c288() -> (w242:T4)  [unwired: 4 in]
        n175 = timed-loop {
          tunnel: w240 -> [w263]
          tunnel: w239 -> [w262]
          timing: w242 -> [_]
          timing-out: [_] -> w241
          shift-right: [w251] -> _
          shift-left: FALSE -> [w254]
          tunnel: [w250] -> w234
          tunnel: [w248] -> w233
          tunnel: [w246] -> w232
          tunnel: w231 -> [w244]
          tunnel: w230 -> [w243]
          stop <- w247 stop-if-true
          # "UDP Broadcast loop"
          n176 = node-c288() -> ()  [unwired: 1 in, 1 out]
          n177 = local read "Flight Number"() -> (w245:string)
          n178 = feedback-in #1(w245) -> ()
          n179 = feedback #1() -> (w256:string)  [unwired: 1 in]
          n180 = Not Equal?(x=w245, y=w256) -> (x != y?=w255:bool)
          n181 = String To IP(1:"239.1.4.6" ("name")) -> (0:w260:u32)
          n182 = flat-sequence {
            tunnel: w260 -> [w270]
            tunnel: w262 -> [w271]
            tunnel: w263 -> [w272]
            tunnel: [w272] -> w259
            tunnel: [w271] -> w258
            tunnel: [w270] -> w257
            tunnel: w255 -> [w269]
            tunnel: u16 50001 ("port or service name") -> [w283]
            tunnel: w259 -> [w282]
            tunnel: w258 -> [w281]
            tunnel: w257 -> [w280]
            tunnel: [w279] -> w250
            tunnel: [w278] -> w248
            tunnel: w244 -> [w276]
            tunnel: w243 -> [w275]
            frame #0 {
              n183 = feedback #2(u32 0) -> (w266:u32)
              n184 = case shown="False" w269 {
                tunnel: w266 -> [w273 _]
                tunnel: [w273 u32 0] -> w265
                frame False {
                }
                frame True {
                }
              }
              "UDP_Pack_num" <- w265
              n185 = Increment(x=w265) -> (x+1=w267:u32)
              n186 = feedback-in #2(w267) -> ()
            }
            frame #1 {
              n187 = Dequeue Element(queue=w276, error in (no error)=w275) -> (element=w277:string)  [unwired: 1 in, 3 out]
              n188 = UDP Write(address=w280, port or service name=w283, connection ID=w282, data in=w277, 8:w281) -> (error out=w278:errorcluster, 3:w279:refnum<k16>)  [unwired: 1 in]
            }
          }
          n189 = Select(t=FALSE, s=w254, f=TRUE) -> (s? t:f=w251:bool)
          "UDP_Out Status" <- w251
          n190 = local read "stop"() -> (w246:bool)
          n191 = node-c288() -> ()  [unwired: 1 in, 1 out]
          n192 = Unbundle(w248) -> ("status"=w249:bool)  [unwired: 2 out]
          n193 = Compound Arithmetic op=OR(w249, w246) -> (w247:bool)
        }
        n194 = node-c288(w241) -> ()  [unwired: 1 out]
        n195 = UDP Close(connection ID=w234, 8:w233) -> (error out=→"UDP_Out_Error Out":errorcluster)  [unwired: 1 out]
        n196 = Wait (ms)(milliseconds to wait=u32 1000) -> ()  [unwired: 1 out]
      }
      n197 = while {
        tunnel: w59 -> [w330]
        tunnel: w58 -> [w329]
        stop <- w333 stop-if-true
        # "Must Delay to avoid 100% CPU"
        # "TCP Loop writing to FISH Tank"
        n198 = TCP Open Connection(address="192.168.101.110", remote port or service name=u16 3502) -> (connection ID=w336:refnum<k5>, error out=w331:errorcluster)  [unwired: 3 in]
        n199 = case shown="No Error" w331 {
          selector: w331 -> [w341 w368]
          tunnel: w336 -> [w346 w369]
          tunnel: [w345 w369] -> w335
          tunnel: [w344 w368] -> w334
          tunnel: [w343 w367] -> w333
          tunnel: w330 -> [w340 _]
          tunnel: w329 -> [w339 _]
          frame No Error {
            n200 = node-c288() -> (w348:T4)  [unwired: 4 in]
            n201 = timed-loop {
              tunnel: w346 -> [w362]
              tunnel: w341 -> [w361]
              tunnel: [w360] -> w345
              tunnel: [w359] -> w344
              tunnel: [w351] -> w343
              shift-right: [w353] -> _
              shift-left: FALSE -> [w356]
              timing: w348 -> [_]
              timing-out: [_] -> w347
              tunnel: w340 -> [w350]
              tunnel: w339 -> [w349]
              stop <- w357 stop-if-true
              n202 = node-c288() -> ()  [unwired: 1 in, 1 out]
              n203 = Dequeue Element(queue=w350, error in (no error)=w349) -> (element=w352:string)  [unwired: 1 in, 3 out]
              n204 = Select(t=FALSE, s=w356, f=TRUE) -> (s? t:f=w353:bool)
              "TCP packet\nSend To FISH" <- w353
              n205 = TCP Write(connection ID=w362, data in=w352, error in (no error)=w361) -> (connection ID out=w360:refnum<k5>, error out=w359:errorcluster)  [unwired: 1 in, 1 out]
              n206 = local read "stop"() -> (w351:bool)
              n207 = Unbundle(w359) -> ("status"=w358:bool)  [unwired: 2 out]
              n208 = node-c288() -> ()  [unwired: 1 in, 1 out]
              n209 = Compound Arithmetic op=OR(w358, w351) -> (w357:bool)
            }
            n210 = node-c288(w347) -> ()  [unwired: 1 out]
          }
          frame Error {
            n211 = local read "stop"() -> (w367:bool)
          }
        }
        n212 = TCP Close Connection(connection ID=w335, error in (no error)=w334) -> (error out=→"FISH TCP Error Out":errorcluster)  [unwired: 1 in, 1 out]
        n213 = Wait (ms)(milliseconds to wait=u32 1000) -> ()  [unwired: 1 out]
      }
      n214 = while {
        tunnel: w61 -> [w372]
        tunnel: w60 -> [w371]
        stop <- w375 stop-if-true
        # "Must Delay to avoid 100% CPU"
        # "TCP Loop writing to SEPTIC Tank"
        n215 = TCP Open Connection(address="192.168.101.108", remote port or service name=u16 3502) -> (connection ID=w378:refnum<k5>, error out=w373:errorcluster)  [unwired: 3 in]
        n216 = case shown="No Error" w373 {
          selector: w373 -> [w383 w410]
          tunnel: w378 -> [w388 w411]
          tunnel: [w387 w411] -> w377
          tunnel: [w386 w410] -> w376
          tunnel: [w385 w409] -> w375
          tunnel: w372 -> [w382 _]
          tunnel: w371 -> [w381 _]
          frame No Error {
            n217 = node-c288() -> (w390:T4)  [unwired: 4 in]
            n218 = timed-loop {
              tunnel: w388 -> [w404]
              tunnel: w383 -> [w403]
              tunnel: [w402] -> w387
              tunnel: [w401] -> w386
              tunnel: [w393] -> w385
              shift-right: [w395] -> _
              shift-left: FALSE -> [w398]
              timing: w390 -> [_]
              timing-out: [_] -> w389
              tunnel: w382 -> [w392]
              tunnel: w381 -> [w391]
              stop <- w399 stop-if-true
              n219 = node-c288() -> ()  [unwired: 1 in, 1 out]
              n220 = Dequeue Element(queue=w392, error in (no error)=w391) -> (element=w394:string)  [unwired: 1 in, 3 out]
              n221 = Select(t=FALSE, s=w398, f=TRUE) -> (s? t:f=w395:bool)
              "TCP packet\nSend To SEPTIC" <- w395
              n222 = TCP Write(connection ID=w404, data in=w394, error in (no error)=w403) -> (connection ID out=w402:refnum<k5>, error out=w401:errorcluster)  [unwired: 1 in, 1 out]
              n223 = local read "stop"() -> (w393:bool)
              n224 = Unbundle(w401) -> ("status"=w400:bool)  [unwired: 2 out]
              n225 = node-c288() -> ()  [unwired: 1 in, 1 out]
              n226 = Compound Arithmetic op=OR(w400, w393) -> (w399:bool)
            }
            n227 = node-c288(w389) -> ()  [unwired: 1 out]
          }
          frame Error {
            n228 = local read "stop"() -> (w409:bool)
          }
        }
        n229 = TCP Close Connection(connection ID=w377, error in (no error)=w376) -> (error out=→"SEPTIC TCP Error Out":errorcluster)  [unwired: 1 in, 1 out]
        n230 = Wait (ms)(milliseconds to wait=u32 1000) -> ()  [unwired: 1 out]
      }
    }
    frame Error {
    }
  }
  n231 = VISA Close(VISA resource name=w15, error in (no error)=w16) -> (error out=→"Serial error out":errorcluster)
